vi "Channel_SetupTDMS.vi"(8 "error in (no error)":errorcluster, 9 "Group Name":string, 10 "tdms file in":refnum<k34>, 11 "Channel in":refnum<class "Channel.lvclass">) -> (0 "error out":errorcluster, 2 "tdms file out":refnum<k34>, 3 "Channel out":refnum<class "Channel.lvclass">)   [LabVIEW 2023, in "Channel.lvclass"]
doc: "Create the channel and channel properties in the given TDMS file ref."
uses:
  Channel.lvclass
  Channel.lvclass/Channel.ctl
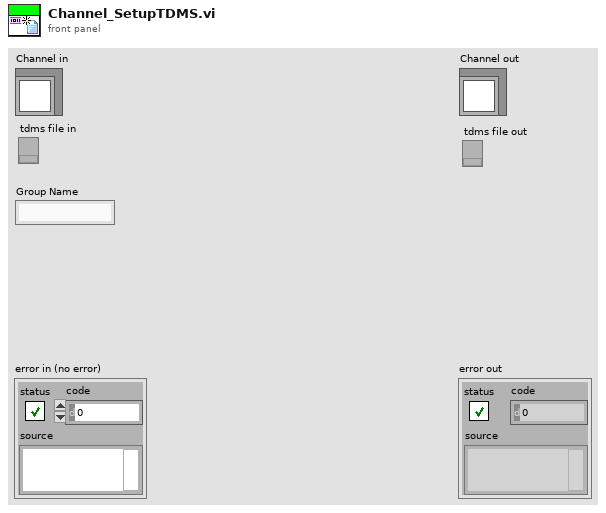
[diagram p1: front panel]
types:
  T1 = typedef "Meta Data.ctl" = cluster{"Key":string, "Value":string}
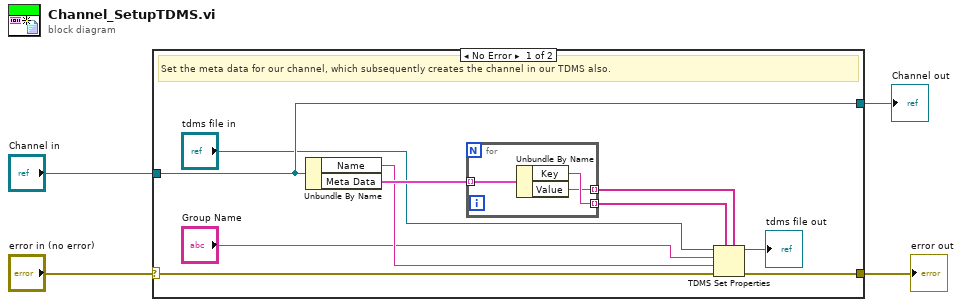
[diagram p0: block diagram]
diagram:
  n1 = case shown="No Error" "error in (no error)" {
    selector: "error in (no error)" -> [w8 w19]
    tunnel: [w9 w19] -> w3
    tunnel: [w13 w18] -> w1
    tunnel: "Channel in" -> [w13 w18]
    frame No Error {
      # "Set the meta data for our channel, which subsequently creates the channel in our TDMS also."
      n2 = Unbundle By Name(w13) -> ("Name"=w12:string, "Meta Data"=w14:T1[])
      n3 = for {
        tunnel: w14 -> [w17] mode=indexing
        tunnel: [w16] -> w6 mode=indexing
        tunnel: [w15] -> w5 mode=indexing
        n4 = Unbundle By Name(w17) -> ("Key"=w16:string, "Value"=w15:string)
      }
      n5 = TDMS Set Properties(5:w5, 7:w6, 8:w8, 9:w12, 10:"Group Name", 11:"tdms file in") -> (0:w9:errorcluster, 3:→"tdms file out":refnum<k34>)  [unwired: 2 out]
    }
    frame Error {
    }
  }
  "error out" <- w3
  "Channel out" <- w1
